vi "Drive_Set.vi"   [LabVIEW 2019]
uses:
  Drive_Cluster.ctl
  Drive_Control_States.ctl
  Drive_Orientation_States.ctl
  <vilib>/Rock Robotics/WPI/DriverStation/WPI_DriverStationRobotMode2.ctl
  Globals/Drive_Globals.vi
  Robot Global Data.vi
panel:
  # "e"
types:
  T1 = typedef "Drive_Cluster.ctl" = cluster{"Control_State":T2, "Vertical_Throttle":dbl, "Lateral_Throttle":dbl, "Rotational_Throttle":dbl, "Strafe_In_Deadband":bool, "Rotation_In_Deadband":bool, "Orientation_State":T3, "Parameters":dbl[], "Step":i32, "Auto_Notifier":refnum<notifier>, "PathName":string}
  T2 = typedef "Drive_Control_States.ctl" = enum16{"No-Op", "Manual_Control", "Command_DriveDistanceAtAngle", "Command_DrivePath"}
  T3 = typedef "Drive_Orientation_States.ctl" = enum16{"Robot-Oriented", "Field-Oriented"}
  T4 = typedef "WPI_DriverStationRobotMode2.ctl" = enum16{"Autonomous Disabled", "Autonomous Enabled", "Teleop Disabled", "Teleop Enabled", "Disconnected", "Finish", "Test Disabled", "Test Enabled", "Emergency Stopped"}
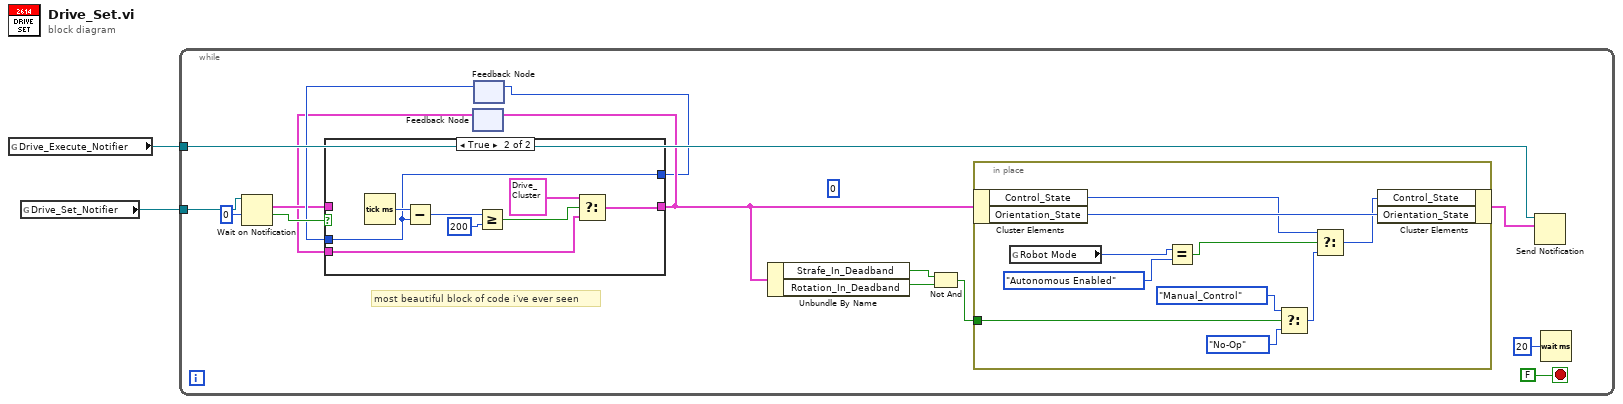
[diagram p0: block diagram]
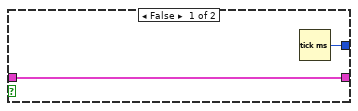
[diagram p2: hidden frame]
diagram:
  n1 = global read "Drive_Globals.vi" "Drive_Execute_Notifier"() -> (w2:refnum<notifier>)
  n2 = global read "Drive_Globals.vi" "Drive_Set_Notifier"() -> (w1:refnum<notifier>)
  n3 = while {
    tunnel: w2 -> [w14]
    tunnel: w1 -> [w15]
    stop <- FALSE stop-if-true
    (unwired) 0 ("timeout in ms (-1)")
    # "most beautiful block of code i've ever seen"
    n4 = Wait on Notification(notifier=w15, timeout in ms (-1)=0) -> (notification=w4:T1, timed out?=w8:bool)  [unwired: 2 in, 2 out]
    n5 = feedback #1() -> (w3:T1)  [unwired: 1 in]
    n6 = feedback #2() -> (w5:u32)  [unwired: 1 in]
    n7 = case shown="True" w8 {
      tunnel: w4 -> [w19 _]
      tunnel: [w19 w27] -> w7
      tunnel: w3 -> [_ w26]
      tunnel: [w18 w24] -> w6
      tunnel: w5 -> [_ w24]
      frame False {
        n8 = Tick Count (ms)() -> (millisecond timer value=w18:u32)
      }
      frame True {
        n9 = Tick Count (ms)() -> (millisecond timer value=w25:u32)
        n10 = Subtract(x=w25, y=w24) -> (x-y=w22:u32)
        n11 = Greater Or Equal?(x=w22, y=u32 200) -> (x >= y?=w23:bool)
        n12 = Select(t=T1 {"Control_State"=enum."Manual_Control", "Vertical_Throttle"=0.0, "Lateral_Throttle"=0.0, "Rotational_Throttle"=0.0, "Strafe_In_Deadband"=FALSE, "Rotation_In_Deadband"=FALSE, "Orientation_State"=enum."Robot-Oriented", "Parameters"=[], "Step"=0, "Auto_Notifier"=refnum, "PathName"=""} ("Cluster"), s=w23, f=w26) -> (s? t:f=w27:T1)
      }
    }
    n13 = feedback-in #1(w7) -> ()
    n14 = feedback-in #2(w6) -> ()
    n15 = Unbundle By Name(w7) -> ("Strafe_In_Deadband"=w11:bool, "Rotation_In_Deadband"=w10:bool)
    n16 = Not And(1:w10, 2:w11) -> (0:w9:bool)
    n17 = in-place {
      in-place-border: w9 -> [w28]
      n18 = in-place-cluster #3(w7) -> ("Control_State"=w32:T2, "Orientation_State"=w37:T3)
      n19 = global read "Robot Global Data.vi" "Robot Mode"() -> (w35:T4)
      n20 = Equal?(x=w35, y=WPI_DriverStationRobotMode2."Autonomous Enabled" ("Robot Mode")) -> (x = y?=w34:bool)
      n21 = Select(t=Drive_Control_States."Manual_Control" ("Control_State"), s=w28, f=Drive_Control_States."No-Op" ("Control_State")) -> (s? t:f=w29:T2)
      n22 = Select(t=w32, s=w34, f=w29) -> (s? t:f=w33:T2)
      n23 = in-place-cluster #3("Control_State"=w33, "Orientation_State"=w37) -> (w13:T1)
    }
    n24 = Send Notification(notification=w13, notifier=w14) -> ()  [unwired: 1 in, 2 out]
    n25 = Wait (ms)(milliseconds to wait=u32 20) -> ()  [unwired: 1 out]
  }
